vi "send_error.vi"(5 "force submission? (F)":bool, 6 "last error? (F)":bool, 7 "additional message":string, 8 "error in (no error)":errorcluster) -> (0 "error out":errorcluster)   [LabVIEW 2010, in "ErrorController.lvclass"]
uses:
  ErrorController.lvclass
  error_cluster.ctl
  class_data.vi
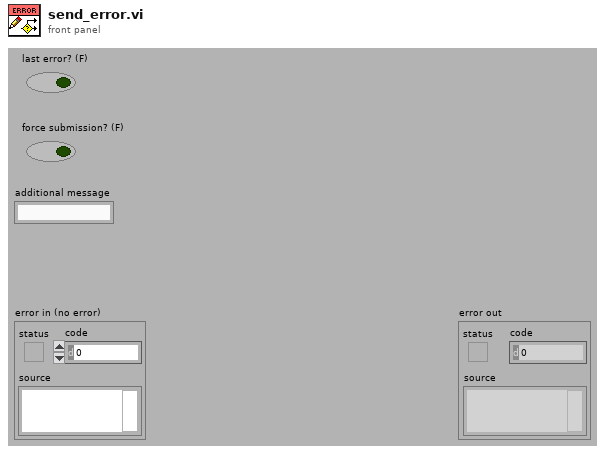
[diagram p1: front panel]
types:
  T1 = typedef "ErrorController.lvclass/error_cluster.ctl" = cluster{"error out":errorcluster, "call chain":string[], "additional message":string, "terminate?":bool, "concatenated string":string}
  T2 = typedef "ErrorController.lvclass/queue controller.ctl" = refnum<queue>
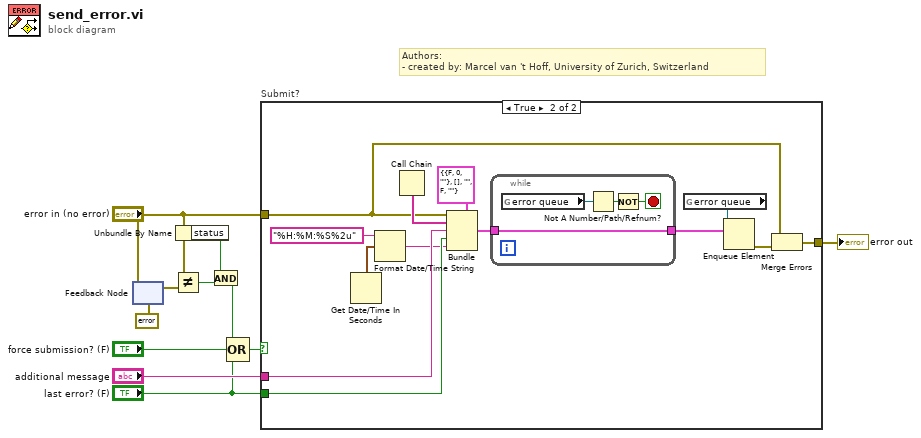
[diagram p0: block diagram]
diagram:
  # "Authors: \n- created by: Marcel van 't Hoff, University of Zurich, Switzerland"
  n1 = feedback #1(errorcluster {"status"=FALSE, "code"=0, "source"=""} ("error IO")) -> (w8:errorcluster)
  n2 = feedback-in #1("error in (no error)") -> ()
  n3 = Not Equal?(x="error in (no error)", y=w8) -> (x != y?=w4:bool)
  n4 = Unbundle By Name("error in (no error)") -> ("status"=w2:bool)
  n5 = And(x=w2, y=w4) -> (x .and. y?=w1:bool)
  n6 = Compound Arithmetic op=OR(w1, "force submission? (F)", "last error? (F)") -> (w6:bool)
  n7 = case "Submit?" shown="True" w6 {
    tunnel: [w12 w22] -> w11
    tunnel: "error in (no error)" -> [w12 w14]
    tunnel: "additional message" -> [_ w21]
    tunnel: "last error? (F)" -> [_ w20]
    frame False {
    }
    frame True {
      n8 = Get Date/Time In Seconds() -> (seconds since 1Jan1904=w19:timestamp)
      n9 = Format Date/Time String(time format string (%c)="%H:%M:%S%2u", seconds (now)=w19) -> (date/time string=w17:string)  [unwired: 1 in]
      n10 = Call Chain() -> (call chain=w24:string[])
      n11 = Bundle(cluster=T1 {"error out"={"status"=FALSE, "code"=0, "source"=""}, "call chain"=[], "additional message"="", "terminate?"=FALSE, "concatenated string"=""} ("element"), "error out"=w14, "call chain"=w24, "additional message"=w21, "terminate?"=w20, "concatenated string"=w17) -> (w16:T1)
      n12 = while {
        tunnel: [w29] -> w15
        tunnel: w16 -> [w29]
        stop <- w26 stop-if-true
        n13 = global read "class_data.vi" "error queue"() -> (w28:T2)
        n14 = Not A Number/Path/Refnum?(number/path/refnum=w28) -> (NaN/Path/Refnum?=w27:bool)
        n15 = Not(x=w27) -> (.not. x?=w26:bool)
      }
      n16 = global read "class_data.vi" "error queue"() -> (w25:T2)
      n17 = Enqueue Element(queue=w25, element=w15) -> (error out=w13:errorcluster)  [unwired: 2 in, 2 out]
      n18 = Merge Errors(w14, w13) -> (w22:errorcluster)
    }
  }
  "error out" <- w11
